vi "Error_Helper_RaiseErrorFromLabel.vi"(6 "Additional Info":string, 7 "Raise?":bool, 8 "Error In":errorcluster, 9 "Error Labels":T2) -> (0 "Error Out":errorcluster)   [LabVIEW 2014, in "hse-misc.lvlib"]
doc: "If <b>Raise?</b> is true, sets an error with code set by <b>Error Labels</b> and source by <b>Additional Info</b>\n\n\n____\nHAMPEL SOFTWARE ENGINEERING v0.12.0 (2018-09-13 18:21)"
uses:
  hse-misc.lvlib
  Error_Labels.ctl
  Error_Codes.ctl
panel:
  in  "Error Codes":T1
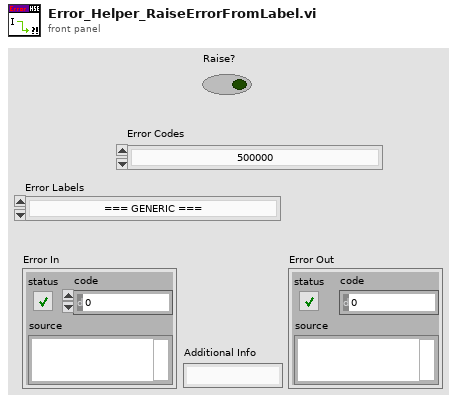
[diagram p1: front panel]
types:
  T1 = typedef "hse-misc.lvlib/Error_Codes.ctl" = enum16{"500000", "500001", "500002", "500003", "500004", "500005", "500006", "500007", "500008", "500009", "500019", "500020", "500021", "500023", "500051", "500052", "500053", "500054", "500055", "500056", "501001", "501002", "501003", "501004", "501005", "510001", "510002", "510056", "510059", "510060", "510200", "510400", "510600", "510601", "520000", "520001", "520002", "520003", "520004", "520005", "520006", "521000", "521200", "550000", "550200"}
  T2 = typedef "hse-misc.lvlib/Error_Labels.ctl" = enum16{"=== GENERIC ===", "Unexpected / unknown error", "Timeout", "Device or resource not found", "Expected (handled) error", "Module or VI not executable", "Server shutting down", "File not found", "Cancelled by user", "Invalid parameter", "Configuration type invalid", "Configuration token not found", "Error occurred parsing configuration string", "External program returned with error", "Unexpected data", "Unknown message", "Attribute not found (in a variant or tree)", "Number of elements mismatch (e.g. in an array)", "Maximum number of attempts (e.g. for a reconnection)", "Input out of range", "Registry file not found or not readable", "Registry type mismatch", "Project name mismatch", "System identifier mismatch", "Configuration file not found", "Checking remote path failed", "Establishing data connection failed", "The network operation exceeded the time limit", "Network is down/unreachable/reset", "The specified port or network address is currently in use", "=== NI DISCOVERY PROTOCOL ===", "=== APPLICATION BUILDER ===", "=== GIT ===", "Return code != 0", "=== FGPA ===", "Generic FPGA error", "Timeout general", "Timeout FIFO", "Timeout DMA", "Timeout Handshake", "Loop time exceeded", "=== IO ===", "=== PROFINET ===", "=== USER INTERFACE ===", "=== GENERIC NETWORKING (NET-TX & NET-RX ==="}
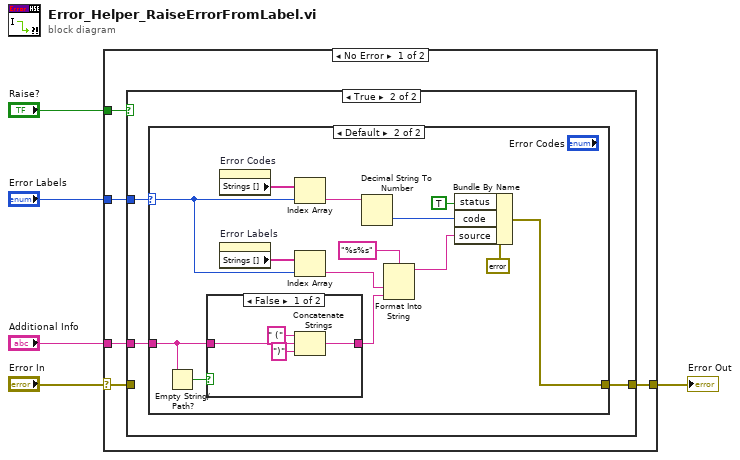
[diagram p0: block diagram]
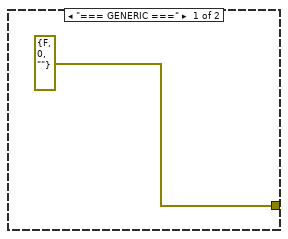
[diagram p3: hidden frame]
diagram:
  n1 = case shown="No Error" "Error In" {
    selector: "Error In" -> [w6 w35]
    tunnel: [w10 w35] -> w5
    tunnel: "Error Labels" -> [w9 _]
    tunnel: "Additional Info" -> [w8 _]
    tunnel: "Raise?" -> [w7 _]
    frame No Error {
      n2 = case shown="True" w7 {
        tunnel: [w11 w14] -> w10
        tunnel: w9 -> [_ w13]
        tunnel: w8 -> [_ w12]
        tunnel: w6 -> [w11 _]
        frame False {
        }
        frame True {
          n3 = case shown="Default" w13 {
            selector: w13 -> [_ w25]
            tunnel: [errorcluster {"status"=FALSE, "code"=0, "source"=""} ("error IO") w29] -> w14
            tunnel: w12 -> [_ w18]
            frame "=== GENERIC ===" {
            }
            frame Default {
              n4 = Empty String/Path?(string/path=w18) -> (empty?=w19:bool)
              n5 = case shown="False" w19 {
                tunnel: w18 -> [w33 w34]
                tunnel: [w32 w34] -> w17
                frame False {
                  n6 = Concatenate Strings(" (" ("string"), w33, ")" ("string")) -> (w32:string)
                }
                frame True {
                }
              }
              n7 = property on="Error Codes" class="Enum (strict)"() -> ("Strings []"=w16:string[])  [unwired: 2 in, 2 out]
              n8 = property on="Error Labels" class="Enum (strict)"() -> ("Strings []"=w26:string[])  [unwired: 2 in, 2 out]
              n9 = Index Array(array=w16, index=w25) -> (element=w24:string)
              n10 = Index Array(array=w26, index=w25) -> (element=w20:string)
              n11 = Decimal String To Number(string=w24) -> (number=w23:i32)  [unwired: 2 in, 1 out]
              n12 = Format Into String(format string="%s%s", w20, w17) -> (resulting string=w22:string)  [unwired: 2 in, 1 out]
              n13 = Bundle By Name(cluster=errorcluster {"status"=TRUE, "code"=0, "source"=""} ("error IO"), "status"=TRUE, "code"=w23, "source"=w22) -> (w29:errorcluster)
            }
          }
        }
      }
    }
    frame Error {
    }
  }
  "Error Out" <- w5
